vi "Start Camera.vi"(8 "error in (no error)":errorcluster, 9 "Config file":path, 10 "IMAQdx Session":T1, 11 "Camera Tester in":refnum<class "Camera Tester.lvclass">) -> (0 "error out":errorcluster, 3 "Camera Tester out":refnum<class "Camera Tester.lvclass">)   [LabVIEW 2014, in "Camera Tester.lvlib" / "Camera Tester.lvclass"]
uses:
  Camera Tester.lvclass
  <vilib>/userdefined/High Color/IMAQdx.ctl
  IMAQdx Actor/IMAQdx Actor/IMAQdx Actor.lvclass
  Logbook/SysLogbook/SysLogbook.lvclass
  Camera Tester Messages/New image Msg/New image Msg.lvclass
  <vilib>/ActorFramework/Actor/Actor.lvclass/Actor.ctl
  <vilib>/ActorFramework/Message Enqueuer/Message Enqueuer.lvclass/Message Enqueuer.ctl
  Camera Tester.lvclass/Camera Tester.ctl
  Logbook/SysLogbook/SysLogbook.lvclass/SysLogbook.ctl
  Camera Actor/Camera Actor/Camera Actor.lvclass/Camera Actor.ctl
  Camera Actor/Camera Actor Messages/Start Acquisition Msg/Start Acquisition Msg.lvclass/Start Acquisition Msg.ctl
  Logbook/SysLogbook/Write Device name.vi
  Logbook/SysLogbook/Write Config file.vi
  Camera Actor/Camera Actor/Write Camera Name.vi
  Camera Actor/Camera Actor/Write Image Receiver.vi
  Camera Actor/Camera Actor/Write Msg Logger.vi
  Camera Actor/Camera Actor/Write New Image Msg.vi
  <vilib>/ActorFramework/Message Enqueuer/Enqueue.vi
  <vilib>/ActorFramework/Message Enqueuer/Init from Existing Queue.vi
  <vilib>/ActorFramework/Message Priority Queue/Priority Enqueue.vi
  <vilib>/ActorFramework/Message Enqueuer/Message Enqueuer.lvclass
  <vilib>/ActorFramework/Stop Msg/Stop Msg.lvclass
  Camera Actor/Camera Actor Messages/Start Acquisition Msg/Start Acquisition Msg.lvclass
  <vilib>/ActorFramework/Actor/Actor.lvclass
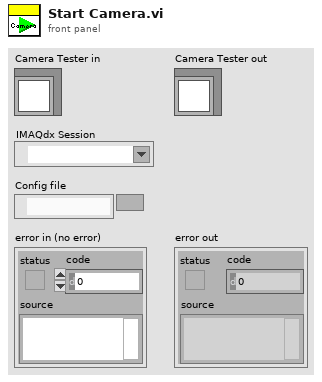
[diagram p1: front panel]
types:
  T1 = typedef "IMAQdx.ctl" = refnum<k21>
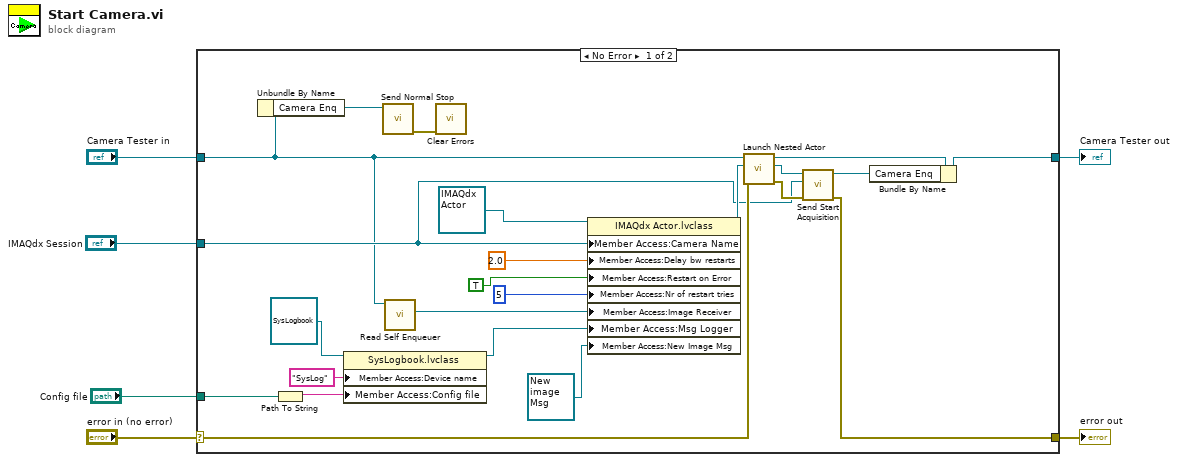
[diagram p0: block diagram]
diagram:
  n1 = case shown="No Error" "error in (no error)" {
    selector: "error in (no error)" -> [w15 w31]
    tunnel: [w12 w31] -> w5
    tunnel: [w17 w30] -> w3
    tunnel: "Camera Tester in" -> [w9 w30]
    tunnel: "IMAQdx Session" -> [w10 _]
    tunnel: "Config file" -> [w21 _]
    frame No Error {
      n2 = Unbundle By Name(w9) -> ("Camera Enq"=w8:refnum<class "Message Enqueuer.lvclass">)
      n3 = Path To String(path=w21) -> (string=w19:string)
      n4 = property class="SysLogbook.lvclass"(reference=refnum<class "SysLogbook.lvclass"> refnum ("SysLogbook.lvclass"), "Member Access:Device name"="SysLog" ("Device name"), "Member Access:Config file"=w19) -> (reference out=w18:refnum<class "SysLogbook.lvclass">)  [unwired: 1 in, 1 out]
      n5 = call <vilib>:"Send Normal Stop.vi"("Message Enqueuer"=w8) -> ("error out"=w7:errorcluster)  [unwired: 10 in]
      n6 = call <vilib>:"Read Self Enqueuer.vi"("Actor"=w9) -> ("Self Enqueuer"=w24:refnum<class "Message Enqueuer.lvclass">)  [unwired: 10 in]
      n7 = call <vilib>:"Clear Errors.vi"("error in (no error)"=w7) -> ()  [unwired: 5 in, 2 out]
      n8 = property class="IMAQdx Actor.lvclass"(reference=refnum<class "IMAQdx Actor.lvclass"> refnum ("IMAQdx Actor.lvlib:IMAQdx Actor.lvclass"), "Member Access:Camera Name"=w10, "Member Access:Delay bw restarts"=dbl[unit] 2.0 ("Delay bw restarts"), "Member Access:Restart on Error"=TRUE ("Restart on Error"), "Member Access:Nr of restart tries"=u8 5 ("Nr of restart tries"), "Member Access:Image Receiver"=w24, "Member Access:Msg Logger"=w18, "Member Access:New Image Msg"=refnum<class "New image Msg.lvclass"> refnum ("Camera Tester.lvlib:New image Msg.lvclass")) -> (reference out=w27:refnum<class "IMAQdx Actor.lvclass">)  [unwired: 1 in, 1 out]
      n9 = call <vilib>:"Launch Nested Actor.vi"("error in (no error)"=w15, "Nested Actor"=w27, "Caller Actor in"=w9) -> ("error out"=w13:errorcluster, "Nested Actor's Enqueuer"=w16:refnum<class "Message Enqueuer.lvclass">, "Caller Actor out"=w29:refnum<class "Camera Tester.lvclass">)  [unwired: 6 in]
      n10 = call "Send Start Acquisition.vi"("error in (no error)"=w13, "Camera Name"=w10, "Message Enqueuer"=w16) -> ("error out"=w12:errorcluster, "Message Enqueuer out"=w14:refnum<class "Message Enqueuer.lvclass">)  [unwired: 7 in]
      n11 = Bundle By Name(cluster=w29, "Camera Enq"=w14) -> (w17:refnum<class "Camera Tester.lvclass">)
    }
    frame Error {
    }
  }
  "error out" <- w5
  "Camera Tester out" <- w3
